vi "reset sesion.vi"(8 "error in (no error)":errorcluster, 11 "5785_2_x_1600MHz in":refnum<class "5785_2_x_1600MHz.lvclass">) -> (0 "error out":errorcluster, 3 "5785_2_x_1600MHz out":refnum<class "5785_2_x_1600MHz.lvclass">)   [LabVIEW 2021, in "5785_2_x_1600MHz.lvclass"]
uses:
  5785_2_x_1600MHz.lvclass
  5785_2_x_1600MHz.lvclass/5785_2_x_1600MHz.ctl
  <vilib>/rvi/interface/nirviReadWriteControl/nirviReadWriteControl.xnode
  <vilib>/rvi/interface/nirviMethod/nirviMethod.xnode
  <vilib>/rvi/errors/niLvFpgaMergeErrorWithErrorCode.vi
  <vilib>/FPGAPlugInAG/Dynamic/niLvFpga_StartFifo_Dynamic.vi
  <vilib>/FPGAPlugInAG/Dynamic/niLvFpga_StopFifo_Dynamic.vi
  NiFpgaLv.dll
  <vilib>/Utility/error.llb/Error Cluster From Error Code.vi
  <vilib>/rvi/interface/Simulation/niFpgaSimulationCallBeginRW.vi
  <vilib>/rvi/errors/niLvFpgaAdjustHostInterfaceError.vi
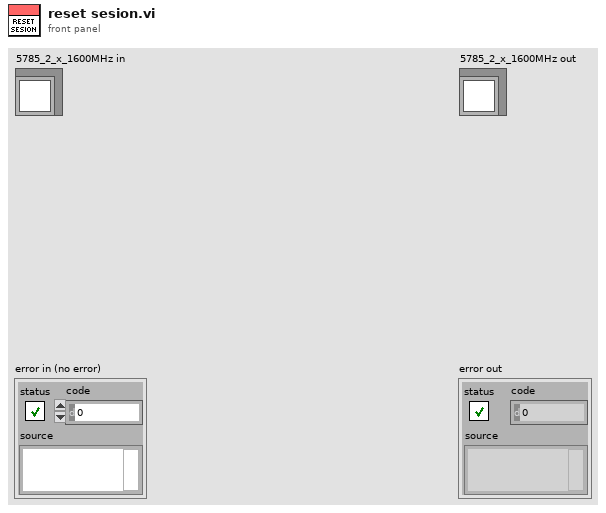
[diagram p1: front panel]
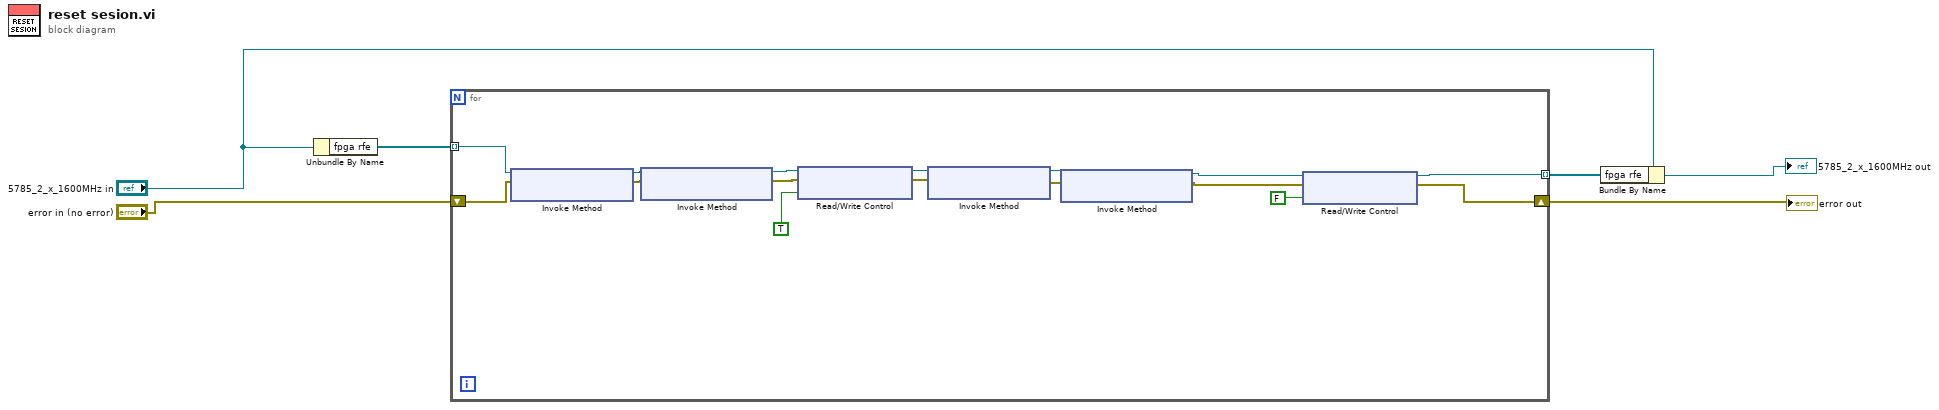
[diagram p0: block diagram]
diagram:
  n1 = Unbundle By Name("5785_2_x_1600MHz in") -> ("fpga rfe"=w6:refnum<k20>[])
  n2 = for {
    tunnel: w6 -> [w19] mode=indexing
    shift-right: [w20] -> w2
    shift-left: "error in (no error)" -> [w16]
    tunnel: [w21] -> w5 mode=indexing
    n3 = xnode "Invoke Method"("FPGA VI Reference In"=w19, "error in"=w16) -> ("FPGA VI Reference Out"=w17:refnum<k20>, "error out"=w18:errorcluster)
    n4 = xnode "Invoke Method"("FPGA VI Reference In"=w17, "error in"=w18) -> ("FPGA VI Reference Out"=w11:refnum<k20>, "error out"=w12:errorcluster)
    n5 = xnode "Read/Write Control"("FPGA VI Reference In"=w11, "error in"=w12, "reset system clock"=TRUE) -> ("FPGA VI Reference Out"=w10:refnum<k20>, "error out"=w9:errorcluster)
    n6 = xnode "Invoke Method"("FPGA VI Reference In"=w10, "error in"=w9) -> ("FPGA VI Reference Out"=w8:refnum<k20>, "error out"=w7:errorcluster)
    n7 = xnode "Invoke Method"("FPGA VI Reference In"=w8, "error in"=w7) -> ("FPGA VI Reference Out"=w15:refnum<k20>, "error out"=w14:errorcluster)
    n8 = xnode "Read/Write Control"("FPGA VI Reference In"=w15, "error in"=w14, "reset system clock"=FALSE) -> ("FPGA VI Reference Out"=w21:refnum<k20>, "error out"=w20:errorcluster)
  }
  "error out" <- w2
  n9 = Bundle By Name(cluster="5785_2_x_1600MHz in", "fpga rfe"=w5) -> (→"5785_2_x_1600MHz out":refnum<class "5785_2_x_1600MHz.lvclass">)
